vi "Open FPGA Ref.vi"(8 "error in (no error)":errorcluster, 10 "Bitfile Path":path, 11 "Device address":string) -> (0 "error out":errorcluster, 3 "FPGA Ref out":refnum<k20>)   [LabVIEW 2025, in "I2C Bus Monitor.lvclass"]
uses:
  I2C Bus Monitor.lvclass
  I2C Bus Monitor.lvclass/I2C Bus Monitor.ctl
  <instrlib>/FlexRIO/API/Host/v1/NI FlexRIO API v1.lvlib
  <vilib>/rvi/interface/nirviCloseFPGA/nirviCloseFPGA.xnode
  <vilib>/FPGAPlugInAG/Dynamic/niLvFpga_Close_Dynamic.vi
  Error Global.vi
  I2C Bus Monitor UI/I2C Bus Monitor UI.lvlib
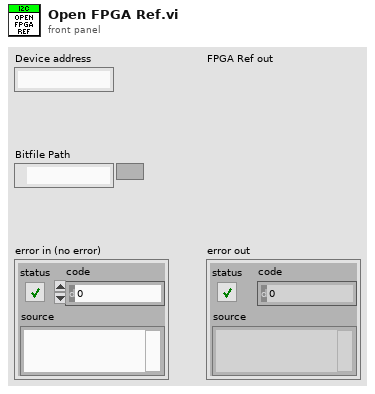
[diagram p1: front panel]
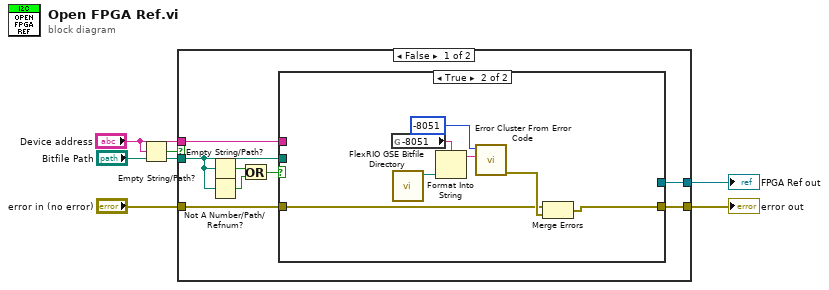
[diagram p0: block diagram]
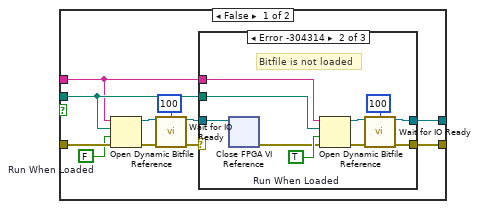
[diagram p2: hidden frame]
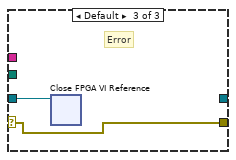
[diagram p4: hidden frame]
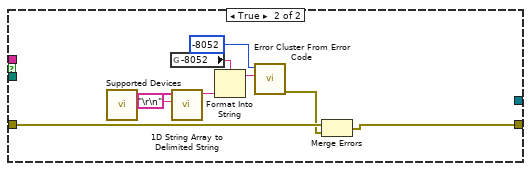
[diagram p5: hidden frame]
diagram:
  n1 = Empty String/Path?(string/path="Device address") -> (empty?=w2:bool)
  n2 = case shown="False" w2 {
    tunnel: [w14 _] -> w6
    tunnel: [w13 w51] -> w5
    tunnel: "Bitfile Path" -> [w8 _]
    tunnel: "Device address" -> [w12 _]
    tunnel: "error in (no error)" -> [w11 w52]
    frame False {
      n3 = Empty String/Path?(string/path=w8) -> (empty?=w9:bool)
      n4 = Not A Number/Path/Refnum?(number/path/refnum=w8) -> (NaN/Path/Refnum?=w10:bool)
      n5 = Or(x=w9, y=w10) -> (x .or. y?=w7:bool)
      n6 = case shown="True" w7 {
        tunnel: [w25 _] -> w14
        tunnel: [w24 w41] -> w13
        tunnel: w8 -> [w23 _]
        tunnel: w12 -> [w22 _]
        tunnel: w11 -> [w19 w42]
        frame False {
          w18 = FALSE  # Run When Loaded
          n7 = Open Dynamic Bitfile Reference(0:w22, 1:w23, 2:w18, 3:w19) -> (5:w16:refnum<k20>, 8:w17:errorcluster)  [unwired: 1 in]
          n8 = call <instrlib>:"Wait for IO Ready.vi"("fpga interface in"=w16, "timeout"=100, "error in"=w17) -> ("fpga interface out"=w21:refnum<k20>, "error out"=w20:errorcluster)  [unwired: 9 in, 2 out]
          n9 = case shown="Error -304314" w20 {
            selector: w20 -> [w27 _ w38]
            tunnel: [w27 w29 w38] -> w24
            tunnel: w21 -> [w26 w37 w39]
            tunnel: w22 -> [_ w31 _]
            tunnel: w23 -> [_ w30 _]
            tunnel: [w26 w28 _] -> w25
            frame No Error {
              # "Bitfile is loaded"
            }
            frame Error {
              w33 = TRUE  # Run When Loaded
              # "Bitfile is not loaded"
              n10 = xnode ("Close FPGA VI Reference")("FPGA VI Reference In"=w37) -> ("error out"=w32:errorcluster)  [unwired: 1 in]
              n11 = Open Dynamic Bitfile Reference(0:w31, 1:w30, 2:w33, 3:w32) -> (5:w35:refnum<k20>, 8:w34:errorcluster)  [unwired: 1 in]
              n12 = call <instrlib>:"Wait for IO Ready.vi"("fpga interface in"=w35, "timeout"=100, "error in"=w34) -> ("fpga interface out"=w28:refnum<k20>, "error out"=w29:errorcluster)  [unwired: 9 in, 2 out]
            }
            frame Default {
              # "Error"
              n13 = xnode ("Close FPGA VI Reference")("FPGA VI Reference In"=w39) -> ()  [unwired: 1 in, 1 out]
            }
          }
        }
        frame True {
          n14 = global read "Error Global.vi" "-8051"() -> (w46:string)
          n15 = call "FlexRIO GSE Bitfile Directory.vi"() -> ("Flexrio GSE Template Bitfiles Folder Path"=w40:path)  [unwired: 11 in]
          n16 = Format Into String(format string=w46, w40) -> (resulting string=w45:string)  [unwired: 2 in, 1 out]
          n17 = call <vilib>:"Error Cluster From Error Code.vi"("error message (\"\")"=w45, "error code (0)"=-8051) -> ("error out"=w43:errorcluster)  [unwired: 7 in]
          n18 = Merge Errors(w42, w43) -> (w41:errorcluster)
        }
      }
    }
    frame True {
      n19 = call "Supported Devices.vi"() -> ("Supported Devices"=w48:string[])  [unwired: 11 in]
      n20 = global read "Error Global.vi" "-8052"() -> (w55:string)
      n21 = call <vilib>:"1D String Array to Delimited String.vi"("delimiter"="\r\n", "string array"=w48) -> ("delimited string"=w47:string)  [unwired: 9 in]
      n22 = Format Into String(format string=w55, w47) -> (resulting string=w54:string)  [unwired: 2 in, 1 out]
      n23 = call <vilib>:"Error Cluster From Error Code.vi"("error message (\"\")"=w54, "error code (0)"=-8052) -> ("error out"=w50:errorcluster)  [unwired: 7 in]
      n24 = Merge Errors(w52, w50) -> (w51:errorcluster)
    }
  }
  "FPGA Ref out" <- w6
  "error out" <- w5
